vi "Memory.Pointer.Read.Unsafe.1D.U64.vi"(8 "error in (no error)":errorcluster, 9 "count":u64 format="%d elements", 10 "buffer in":u64[](array[numeric]), 11 "pointer in":refnum<class "Memory.Pointer.lvclass">) -> (0 "error out":errorcluster, 1 "count out":u64 format="%d elements", 2 "buffer out":u64[](array[numeric]), 3 "pointer out":refnum<class "Memory.Pointer.lvclass">)   [LabVIEW 2016, in "Memory Manager.lvlib" / "Memory.Pointer.lvclass"]
doc: "Reads <b>count</b> elements from the address specified by <b>pointer</b> into the provided <b>buffer</b>.\n\n<b>Note:</b> This VI is <b>unsafe</b>.\n\nUnsafe means that it does not evaluate the size parameter of <b>pointer</b> to ensure that is inbounds of allocated memory before peforming a memory read/write. Reading/writing more data to a pointer than it has allocated can corrupt or crash LabVIEW. Only use this VI in scenarios where the <b>pointer</b> has been validated to be allocated to a correct size before calling this VI."
uses:
  Memory.Pointer.lvclass
  Memory.Pointer.lvclass/Memory.Pointer.ctl
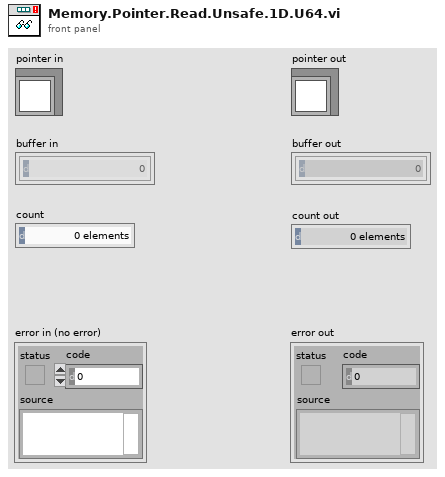
[diagram p1: front panel]
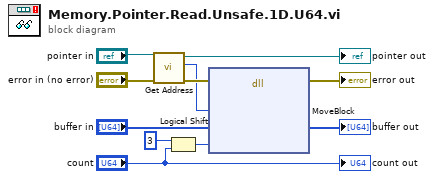
[diagram p0: block diagram]
diagram:
  n1 = call "Get Address.vi"("error in (no error)"="error in (no error)", "Pointer in"="pointer in") -> ("error out"=w11:errorcluster, "address"=w10:u64, "Pointer out"=→"pointer out":refnum<class "Memory.Pointer.lvclass">)  [unwired: 7 in]
  n2 = Logical Shift(y=i16 3, x="count") -> (x << y=w8:u64)
  n3 = dll-call lib="LabVIEW" fn="MoveBlock"(error in=w11, "src"=w10, "dst"="buffer in", "size"=w8) -> (error out=→"error out":errorcluster, "dst"=→"buffer out":u64[])  [unwired: 5 in, 1 out]
  "count out" <- "count"
